vi "audio_crosstalkMeasurement.vi"() -> ()   [LabVIEW 2021, in "audio_crosstalkMeasurement.lvlib"]
uses:
  <vilib>/PDM Acquisition Toolkit/host/Classes/Tasks/PDM Tasks/Controls/Acquisition Mode.ctl
  <vilib>/PDM Acquisition Toolkit/host/Classes/Session/Controls/Logic Levels.ctl
  <vilib>/PDM Acquisition Toolkit/shared/controls/PCM Data Format Configuration.ctl
  <vilib>/PDM Acquisition Toolkit/shared/controls/Digital Edge.ctl
  <vilib>/PDM Acquisition Toolkit/shared/controls/PCM Bit Endianness.ctl
  <vilib>/PDM Acquisition Toolkit/shared/controls/PCM Data Justification.ctl
  <vilib>/PDM Acquisition Toolkit/shared/controls/PCM Frame Sync Control.ctl
  <vilib>/addons/_NISVFA/_Generation/Signal Generation/SV Signal/sv_System Timing Model.ctl
  <vilib>/DAQmx/write.llb/DAQmx Write (Analog 1D Wfm NChan NSamp).vi
  <vilib>/addons/_NISVFA/_Shared subVIs/Common/SVL Set dB Reference (N Ch - 1 Ref).vi
  <vilib>/addons/_NISVFA/_Spectrum Processing/SVFA Unit Conversion (Complex) (1 Ch).vi
  <vilib>/addons/_NISVFA/_Shared subVIs/Common/SVL Set dB Reference (1 Ch).vi
  <vilib>/addons/_NISVFA/_Shared subVIs/Common/svc_Log View for Spectrum (1Ch).vi
  <vilib>/addons/_NISVFA/_Spectrum Processing/SVFA Unit Conversion (1 Ch).vi
  <vilib>/addons/_NISVFA/_Shared subVIs/Common/svc_Complex Datatype Defaults.vi
  <vilib>/addons/_NISVFA/_Shared subVIs/Common/SVL Set dB Reference (variant).vi
  <vilib>/addons/_NISVFA/_Shared subVIs/Common/svc_Unwrap Phase.vi
  <vilib>/addons/_NISVFA/_Shared subVIs/Common/svc_Convert Spectrum Array to dB.vi
  <vilib>/addons/_NISVFA/_Shared subVIs/Common/svc_Spectrum Units.vi
  <vilib>/addons/_NISVFA/_Spectrum Processing/subVIs/svfa_Conversion Utility (spectrum info).vi
  <vilib>/addons/_NISVFA/_Shared subVIs/Common/svc_Format Value (DBL).vi
  <vilib>/addons/_NISVFA/_Shared subVIs/Common/svc_Get Weighting Enum and Labels.vi
  <vilib>/addons/_NISVFA/_Shared subVIs/Common/svc_Engineering Units to Unit Label.vi
  <vilib>/addons/_NISVFA/_Shared subVIs/Common/svc_Surround NonAlpha String with Parentheses.vi
  <vilib>/dlg_ctls.llb/Space Constant.vi
  <vilib>/addons/_NISVFA/_Spectrum Processing/subVIs/svfa_Peak to RMS to Peak2Peak.vi
  <vilib>/addons/_NISVFA/_Spectrum Processing/subVIs/svfa_Mag to Mag2.vi
  <vilib>/addons/_NISVFA/_Spectrum Processing/subVIs/svfa_Linear to dB.vi
  <vilib>/addons/_NISVFA/_Spectrum Processing/subVIs/svfa_dBrefA to dBrefB.vi
  <vilib>/addons/_NISVFA/_Spectrum Processing/subVIs/svfa_Spectrum to Spectral Density.vi
  <vilib>/addons/_NISVFA/_Shared subVIs/Common/svc_Unit Label Lexical Class.vi
  <vilib>/addons/_NISVFA/_Shared subVIs/Common/svc_Window Parameters.vi
  <vilib>/addons/_NISVFA/_Generation/Signal Generation/SV Sinusoid/SV Sinusoid.lvclass
  C:/Program Files/National Instruments/LabVIEW 2021/vi.lib/addons/_NISVFA/_Generation/Signal Generation/SV Signal/SV Signal.lvclass
  <vilib>/DAQmx/create/channels.llb/DAQmx Create Channel (AO-FuncGen).vi
  <vilib>/DAQmx/create/channels.llb/DAQmx Create Channel (AO-Voltage-Basic).vi
  <vilib>/DAQmx/configure/timing.llb/DAQmx Timing (Sample Clock).vi
  <vilib>/addons/_NISVFA/_Generation/Signal Generation/SV Sinusoid/Configure Sine.vi
  <vilib>/addons/_NISVFA/_Generation/Signal Generation/SV Signal/Write Sample Rate.vi
  <vilib>/addons/_NISVFA/_Generation/Signal Generation/SV Signal/Write System Timing Model.vi
  <vilib>/addons/_NISVFA/_Generation/Signal Generation/SV Signal/Write Ramp Parameters.vi
  <vilib>/DAQmx/miscellaneous.llb/DAQmx Fill In Error Info.vi
  <vilib>/PDM Acquisition Toolkit/host/API/Public/Create Tasks/Create PCM Input Task.vi
  <vilib>/PDM Acquisition Toolkit/host/API/Public/Configure/Timing/Configure Timing - PCM Input Slave.vi
  <vilib>/PDM Acquisition Toolkit/host/API/Public/Configure/PDM Channel/Configure Microphone Sensitivity FSPA - PCM Input Task.vi
  <vilib>/PDM Acquisition Toolkit/host/API/Public/Start/Start PCM Input Task.vi
  <vilib>/PDM Acquisition Toolkit/host/API/Public/Read/Read PCM Input Waveform.vi
  <vilib>/addons/_NISVFA/_Shared subVIs/Common/svc_Caller VI Returned in Error Source.vi
  <vilib>/addons/Sound and Vibration/svt_Single Tone Measurements/SVT Crosstalk (Time).vi
  <vilib>/Analysis/4window.llb/window parameters.vi
  <vilib>/Analysis/4window.llb/Window Properties.vi
  <vilib>/Analysis/4window.llb/Window Properties by Name.vi
  <vilib>/PDM Acquisition Toolkit/host/API/Public/Clear/Clear PCM Input Task.vi
  audio_crosstalkMeasurement.lvlib
  <vilib>/addons/Sound and Vibration/svt_Single Tone Measurements/SoundVib_SingleTone.lvlib
  <vilib>/PDM Acquisition Toolkit/host/API/PDM Acquisition Toolkit.lvlib
  <vilib>/PDM Acquisition Toolkit/host/Classes/Tasks/PDM Tasks/PDM Task.lvclass
  <vilib>/PDM Acquisition Toolkit/host/Classes/Session/DecoderSession.lvclass
  <resource>/objmgr/daqmx.rc
  <vilib>/addons/_NISVFA/_Generation/Signal Generation/SV Signal/SV Signal.lvclass
  <vilib>/PDM Acquisition Toolkit/shared/PDM Shared.lvlib
panel:
  in  "Tab Control 2":enum32{"Frequency Domain", "Time Domain"}(tab)=enum."Time Domain"
  out "Spectrum":cluster{"x0":dbl, "dx":dbl, "magnitude":dbl[]}[](graph)
  out "crosstalk":dbl=nan format="%.2f"
  out "Waveform Graph":waveform(dbl)[](graph)
  in  "Tab Control":T1(tab)=enum."Digital Interface"
  in  "Resource name":tag="4468/ao0"
  in  "Frequency":dbl=1000.0 format="%#_6pHz"
  in  "Amplitude":dbl=1.0
  in  "channel list":string="7820\\PCMi 0"
  in  "Sensitivity":dbl=0.34762 format="%#_gFS/Pa"
  in  "Number of words":i32=19200
  in  "Clock rate":u32=12288000 format="%.4pHz"
  in  "Interferer channel":i32
  in  "Victim channel":i32=1
  out "error out":errorcluster
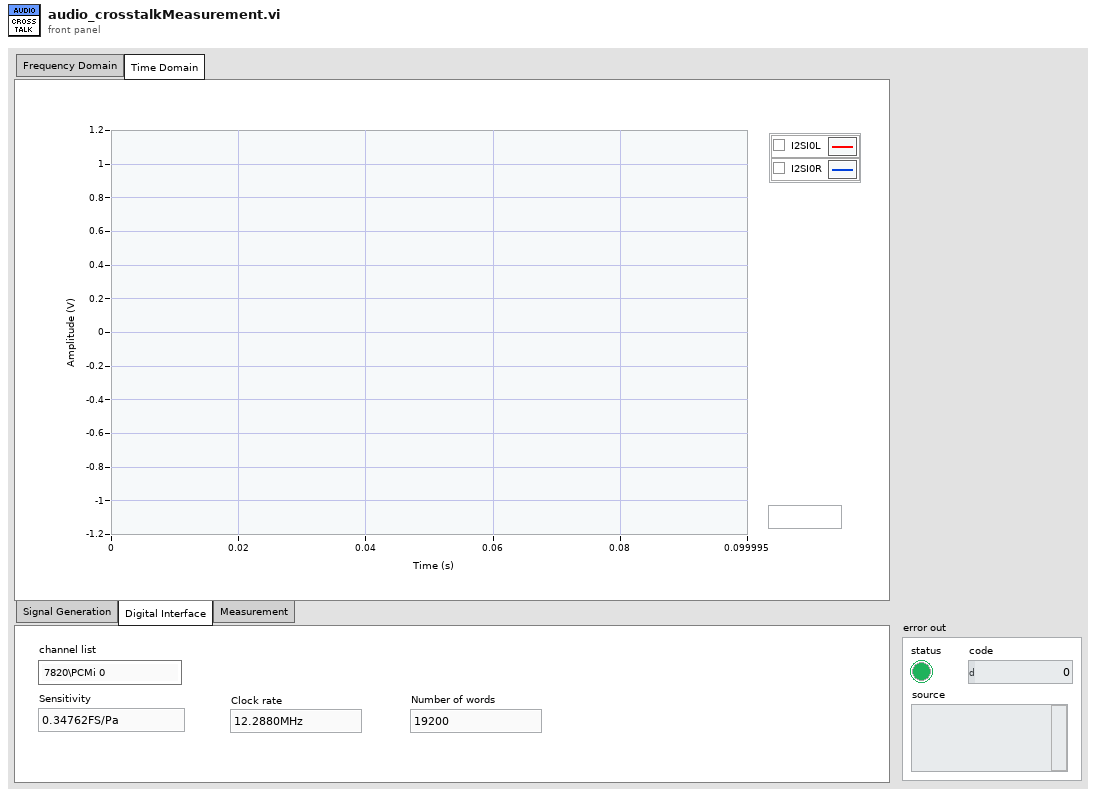
[diagram p1: front panel]
types:
  T1 = enum32{"Signal Generation", "Digital Interface", "Measurement"}
  T2 = typedef "PDM Shared.lvlib/PCM Frame Sync Control.ctl" = cluster{"Frame Length":u16, "Frame Sync Pulse Width":u16, "Bit Clock Edge  Sync":T3}
  T3 = typedef "PDM Shared.lvlib/Digital Edge.ctl" = enum8{"Rising", "Falling"}
  T4 = typedef "PDM Shared.lvlib/PCM Data Format Configuration.ctl" = cluster{"Frame Sync Edge for Channel 0":T3, "Channel Count Per Frame":u8, "Channel Length":u16, "Bit Depth":u8, "Channel 0 Offset":u16, "Endianness":T5, "Data Justification":T6}
  T5 = typedef "PDM Shared.lvlib/PCM Bit Endianness.ctl" = enum16{"MSB First", "LSB First"}
  T6 = typedef "PDM Shared.lvlib/PCM Data Justification.ctl" = enum16{"Left Justified", "Right Justified"}
  T7 = typedef "PDM Acquisition Class Library.lvlib/DecoderSession.lvclass/Logic Levels.ctl" = enum16{"3.3 V", "1.8 V", "1.2 V"}
  T8 = typedef "PDM Acquisition Class Library.lvlib/PDM Task.lvclass/Acquisition Mode.ctl" = enum16{"Finite", "Continuous"}
  T9 = cluster{"linear/dB":enum16{"no change", "linear", "dB"}, "dB reference (0: no change)":dbl, "power/magnitude":enum16{"no change", "power", "magnitude"}, "view":enum16{"no change", "rms", "peak", "peak-peak"}}
  T10 = cluster{"profile":enum16{"Linear", "Half cosine"}, "durations [s]":cluster{"ramp-up":dbl, "transition":dbl, "ramp-down":dbl}}
  T11 = typedef "SV Signal.lvclass/sv_System Timing Model.ctl" = i64
  T12 = typedef "PDM Acquisition Class Library.lvlib/PCM Input Task.lvclass/DVR PCM Input Task.ctl" = refnum<data-value>
  T13 = typedef "svc_Spectrum Info.ctl" = cluster{"channel name":string, "description":string, "x-axis units":T14, "spectral info":cluster{"spectrum type":T15, "linear/dB":enum16{"linear", "dB"}, "window":u16, "window size":i32, "FFT size":i32}, "engineering units":T16, "custom label":string, "dB reference [EU]":dbl, "peak units":enum16{"rms", "peak", "peak-peak"}, "weighting filter":T17, "spectral density?":bool, "unit label":string, "spectrum skewed?":bool, "complimentary spectrum units":T18}
  T14 = typedef "svc_X-Axis Units.ctl" = u16
  T15 = typedef "svc_Spectrum Type.ctl" = enum16{"FFT Spectrum [complex]", "Amplitude [Magnitude]", "Power [Magnitude^2]", "Cross Spectrum [complex]", "Frequency Response [Complex]"}
  T16 = typedef "svc_Engineering Units Text Ring.ctl" = u16
  T17 = typedef "svc_Weighting Filter Text Ring.ctl" = u16
  T18 = typedef "svc_Complimentary Spectrum Units.ctl" = enum16{"none", "radians", "degrees", "cycles", "imaginary"}
  T19 = cluster{"complex spectrum response":cluster{"f0":dbl, "df":dbl, "complex spectrum":cdb[]}, "spectrum info":T13}
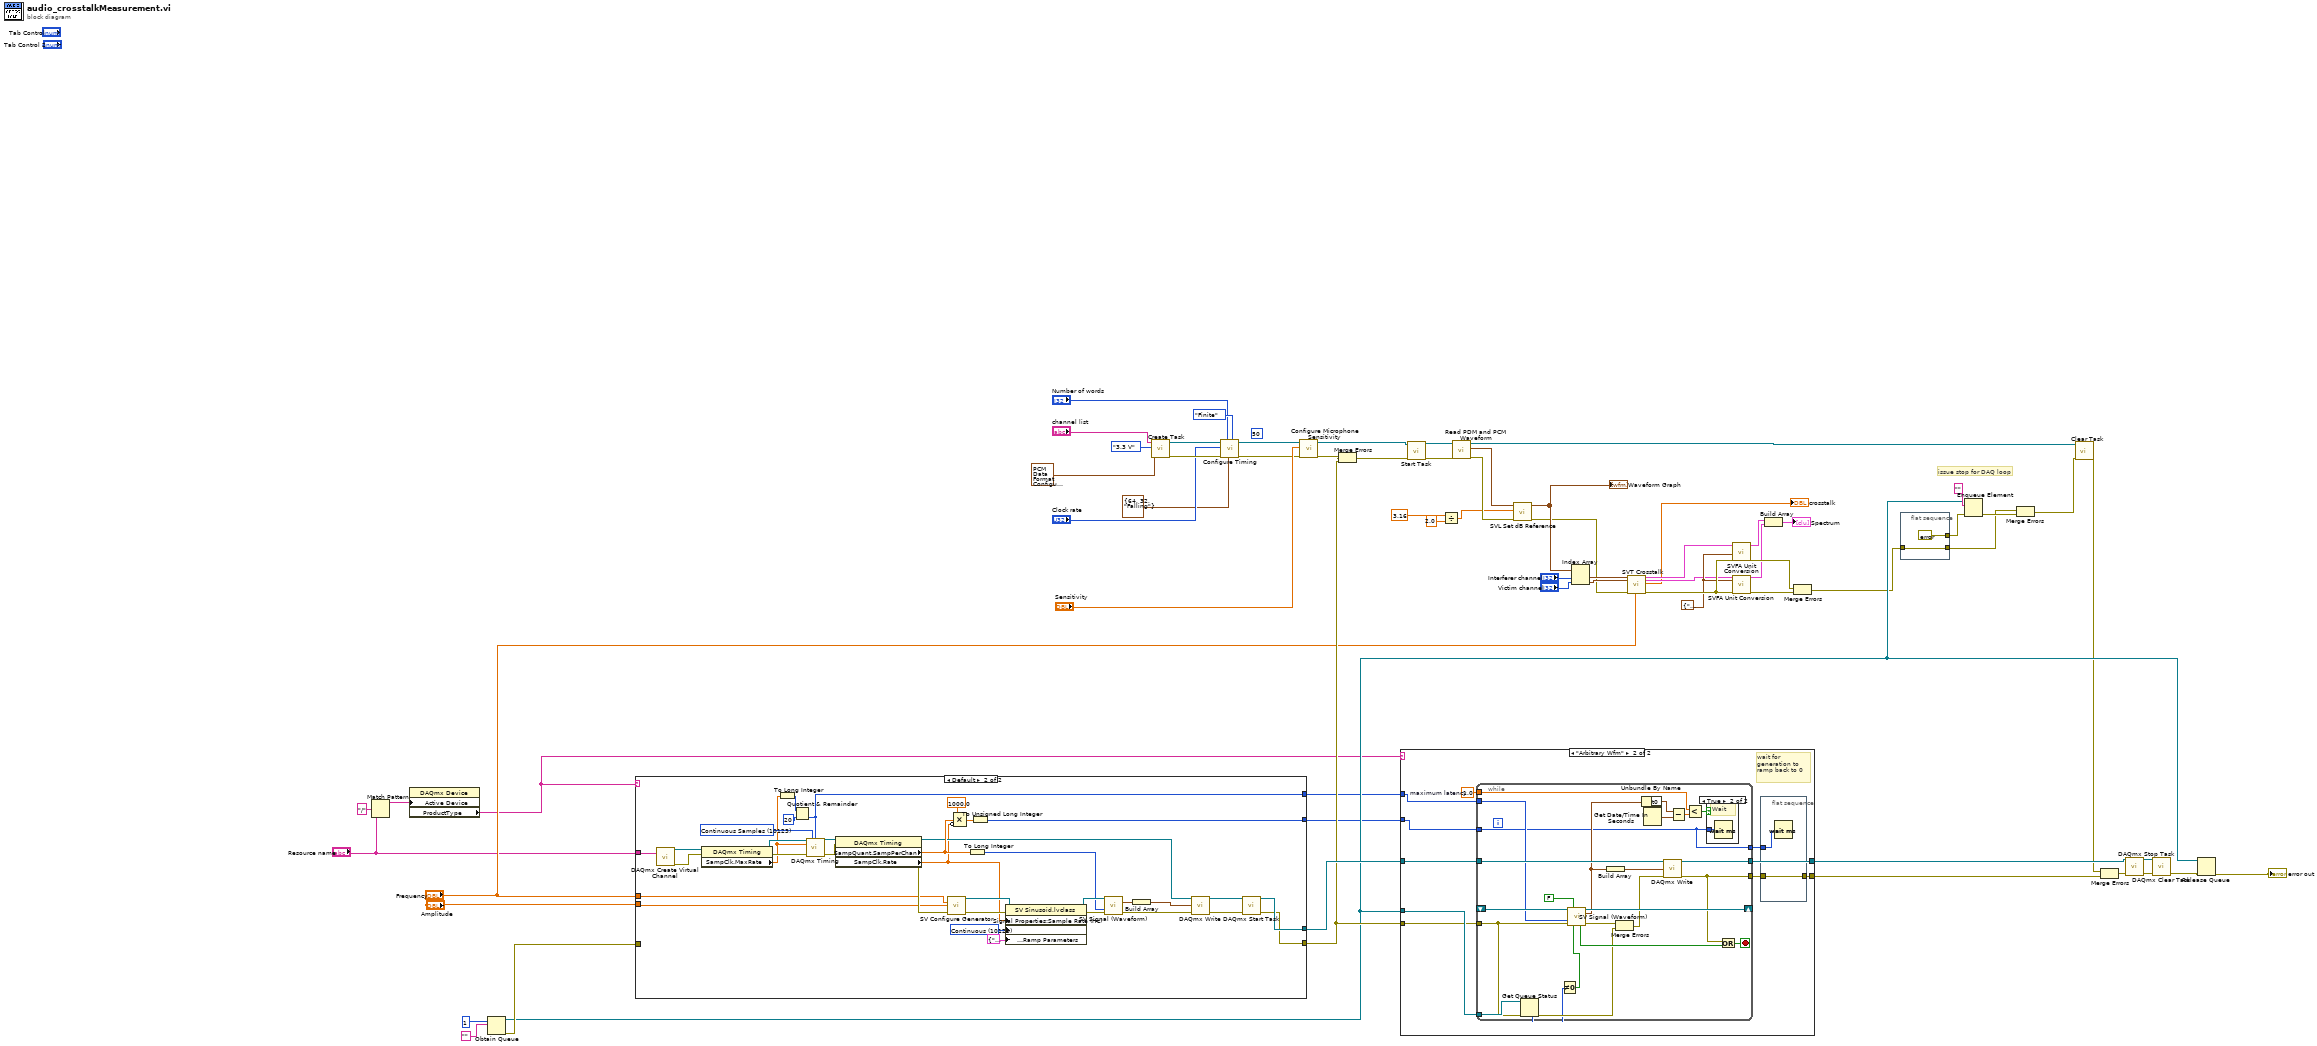
[diagram p0: block diagram]
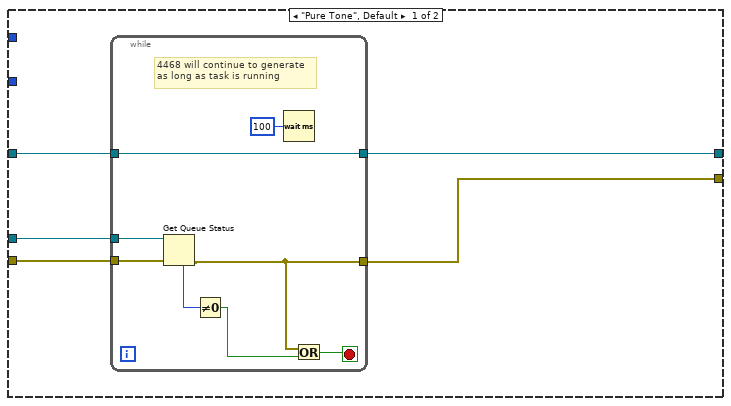
[diagram p2: hidden frame]
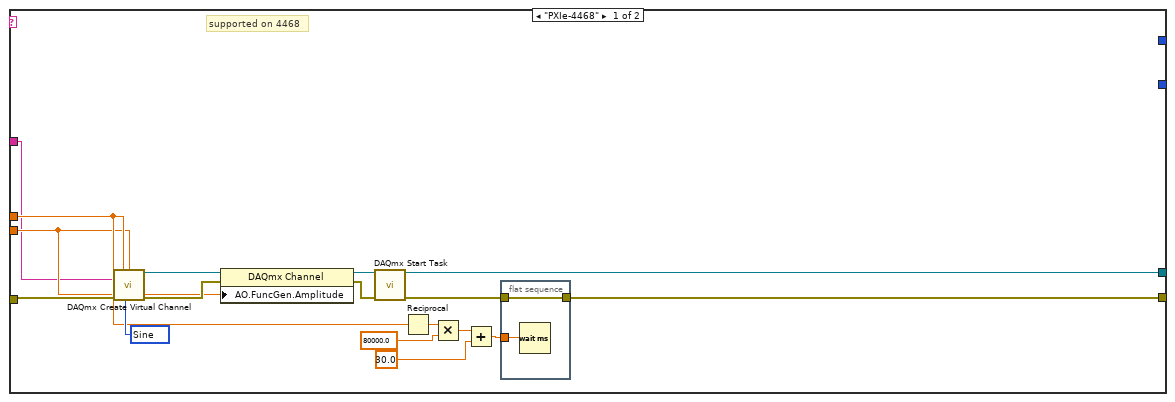
[diagram p4: hidden frame]
diagram:
  (unwired) u8 50 ("data latch at SCK cycle")
  w42 = T9 {"linear/dB"=enum."dB", "dB reference (0: no change)"=0.0, "power/magnitude"=enum."magnitude", "view"=enum."peak"} ("desired scaling")
  # "issue stop for DAQ loop"
  n1 = Match Pattern(string="Resource name", regular expression="/") -> (before substring=w2:string)  [unwired: 1 in, 3 out]
  n2 = property class="DAQmx Device"("Active Device"=w2) -> ("ProductType"=w4:string)  [unwired: 2 in, 2 out]
  n3 = Obtain Queue(max queue size (-1, unlimited)=1, element data type="") -> (queue out=w52:refnum<queue>, error out=w65:errorcluster)  [unwired: 3 in, 1 out]
  n4 = case shown="Default" w4 {
    tunnel: [w72 w93] -> w64
    tunnel: [w71 w92] -> w63
    tunnel: w65 -> [w83 _]
    tunnel: "Frequency" -> [w70 w103]
    tunnel: "Amplitude" -> [w69 w102]
    tunnel: [_ w89] -> w9
    tunnel: [_ w88] -> w10
    tunnel: "Resource name" -> [w68 w87]
    frame "PXIe-4468" {
      w84 = 14751 items=["Sine"=14751, "Triangle"=14752, "Square"=14753, "Sawtooth"=14754] ("type")
      # "supported on 4468"
      n5 = call-poly <vilib>:"DAQmx Create Virtual Channel.vi"("frequency"=w70, "amplitude"=w69, "physical channels"=w68, "type"=w84, "error in"=w83) -> ("task out"=w74:refnum<k21>, "error out"=w73:errorcluster)  [unwired: 9 in]
      n6 = property class="DAQmx Channel"(reference=w74, error in=w73, "AO.FuncGen.Amplitude"=w69) -> (reference out=w76:refnum<k21>, error out=w75:errorcluster)
      n7 = call <vilib>:"DAQmx Start Task.vi"("task/channels in"=w76, "error in"=w75) -> ("task out"=w72:refnum<k21>, "error out"=w82:errorcluster)  [unwired: 12 in]
      n8 = Reciprocal(x=w70) -> (1/x=w81:dbl)
      n9 = Multiply(x=w81, y=80000.0) -> (x*y=w79:dbl)
      n10 = Add(x=w79, y=30.0) -> (x+y=w77:dbl)
      n11 = flat-sequence {
        tunnel: [w86] -> w71
        tunnel: w82 -> [w86]
        tunnel: w77 -> [w85]
        frame #0 {
          n12 = Wait (ms)(milliseconds to wait=w85) -> ()  [unwired: 1 out]
        }
      }
    }
    frame Default {
      w97 = 10123 items=["Finite Samples"=10178, "Continuous Samples"=10123, "Hardware Timed Single Point"=12522] ("sample mode")
      w119 = T11 10123 items=["Finite"=10178, "-"=-1, "Continuous"=10123, "-"=-2, "Settled"=110123, "Averaged"=210123, "Discrete Sweep"=310123, "Continuous Sweep"=410123] ("System Timing Model")
      n13 = call-poly <vilib>:"DAQmx Create Virtual Channel.vi"("physical channels"=w87) -> ("task out"=w98:refnum<k21>, "error out"=w99:errorcluster)  [unwired: 13 in]
      n14 = property class="DAQmx Timing"(reference=w98, error in=w99) -> (reference out=w101:refnum<k21>, error out=w100:errorcluster, "SampClk.MaxRate"=w90:dbl)
      n15 = To Long Integer(number=w90) -> (32bit integer=w91:i32)
      n16 = Quotient & Remainder(x=w91, y=20) -> (floor(x/y)=w89:i32)  [unwired: 1 out]
      n17 = call-poly <vilib>:"DAQmx Timing.vi"("task/channels in"=w101, "sample mode"=w97, "samples per channel"=w89, "rate"=w90, "error in"=w100) -> ("task out"=w95:refnum<k21>, "error out"=w94:errorcluster)  [unwired: 9 in]
      n18 = property class="DAQmx Timing"(reference=w95, error in=w94) -> (reference out=w114:refnum<k21>, error out=w105:errorcluster, "SampQuant.SampPerChan"=w116:dbl, "SampClk.Rate"=w104:dbl)
      n19 = call-poly <vilib>:"SV Configure Generator.vi"("frequency (Hz)"=w103, "amplitude"=w102, "error in (no error)"=w105) -> ("signal configuration"=w120:refnum<class "SV Sinusoid.lvclass">, "error out"=w121:errorcluster)  [unwired: 11 in]
      n20 = Compound Arithmetic op=MULTIPLY(1000.0 ("value"), w116, invert w104) -> (w113:dbl)
      n21 = To Long Integer(number=w116) -> (32bit integer=w115:i32)
      n22 = To Unsigned Long Integer(number=w113) -> (unsigned 32bit integer=w88:u32)
      n23 = property class="SV Sinusoid.lvclass"(reference=w120, error in=w121, "Signal Properties:Sample Rate (Hz)"=w104, "Signal Properties:System Timing Model"=w119, "Signal Properties:Ramps:Ramp Parameters"=T10 {"profile"=enum."Linear", "durations [s]"={"ramp-up"=0.0, "transition"=0.0, "ramp-down"=0.01}} ("Ramp Parameters:All Elements")) -> (reference out=w118:refnum<class "SV Sinusoid.lvclass">, error out=w117:errorcluster)
      n24 = call-dynamic "SV Signal (Waveform).vi"("signal configuration"=w118, "samples"=w115, "error in (no error)"=w117) -> ("output waveform"=w108:waveform(dbl), "error out"=w109:errorcluster)  [unwired: 7 in, 4 out]
      n25 = Build Array(w108) -> (w110:waveform(dbl)[])
      n26 = call-poly <vilib>:"DAQmx Write.vi"("task/channels in"=w114, "data"=w110, "error in"=w109) -> ("task out"=w107:refnum<k21>, "error out"=w106:errorcluster)  [unwired: 10 in, 1 out]
      n27 = call <vilib>:"DAQmx Start Task.vi"("task/channels in"=w107, "error in"=w106) -> ("task out"=w93:refnum<k21>, "error out"=w92:errorcluster)  [unwired: 12 in]
    }
  }
  n28 = call-poly <vilib>:"Create Task.vi"("PCM data configuration"=T4 {"Frame Sync Edge for Channel 0"=enum."Falling", "Channel Count Per Frame"=2, "Channel Length"=32, "Bit Depth"=24, "Channel 0 Offset"=1, "Endianness"=enum."MSB First", "Data Justification"=enum."Left Justified"}, "logic level"=Logic_Levels."3.3 V", "channel list"="channel list") -> ("error out"=w33:errorcluster, "PCM input task out"=w34:T12)  [unwired: 7 in]
  n29 = call-poly <vilib>:"Configure Timing.vi"("acquisition mode"=Acquisition_Mode."Finite", "Frame Sync Clock Control"=T2 {"Frame Length"=64, "Frame Sync Pulse Width"=32, "Bit Clock Edge  Sync"=enum."Falling"}, "number of words per channel"="Number of words", "error in"=w33, "Bit Clock rate"="Clock rate", "PCM input task in"=w34) -> ("error out"=w7:errorcluster, "PCM input task out"=w8:T12)  [unwired: 4 in]
  n30 = call-poly <vilib>:"Configure Microphone Sensitivity.vi"("error in"=w7, "microphone sensitivity (FS/Pa)"="Sensitivity", "PCM input task in"=w8) -> ("error out"=w30:errorcluster, "PCM input task out"=w28:T12)  [unwired: 7 in]
  n31 = Merge Errors(w30, w63) -> (w29:errorcluster)
  n32 = case shown="\"Arbitrary Wfm\"" w4 {
    tunnel: w52 -> [w124 w144]
    tunnel: [w123 w143] -> w60
    tunnel: [w122 w141] -> w12
    tunnel: w64 -> [w126 w140]
    tunnel: w63 -> [w125 w139]
    tunnel: w10 -> [_ w136]
    tunnel: w9 -> [_ w137]
    frame "Pure Tone", Default {
      n33 = while {
        tunnel: w126 -> [w131]
        tunnel: w125 -> [w132]
        tunnel: w124 -> [w133]
        tunnel: [w131] -> w123
        tunnel: [w127] -> w122
        stop <- w130 stop-if-true
        # "4468 will continue to generate as long as task is running"
        n34 = Get Queue Status(queue=w133, error in (no error)=w132) -> (error out=w127:errorcluster, # elements in queue=w134:i32)  [unwired: 1 in, 6 out]
        n35 = Not Equal To 0?(x=w134) -> (x != 0?=w129:bool)
        n36 = Wait (ms)(milliseconds to wait=u32 100) -> ()  [unwired: 1 out]
        n37 = Or(x=w127, y=w129) -> (x .or. y?=w130:bool)
      }
    }
    frame "Arbitrary Wfm" {
      w138 = 1.0  # maximum latency
      # "wait for generation to ramp back to 0"
      n38 = while {
        tunnel: w139 -> [w149]
        shift-right: [w169] -> _
        shift-left: _ -> [w170]
        tunnel: w140 -> [w166]
        tunnel: [w165] -> w143
        tunnel: [w164] -> w142
        tunnel: w138 -> [w160]
        tunnel: w144 -> [w154]
        tunnel: w137 -> [w148]
        tunnel: w136 -> [w147]
        tunnel: [w147] -> w135
        stop <- w168 stop-if-true
        n39 = Get Queue Status(queue=w154, error in (no error)=w149) -> (error out=w152:errorcluster, # elements in queue=w151:i32)  [unwired: 1 in, 6 out]
        n40 = Not Equal To 0?(x=w151) -> (x != 0?=w153:bool)
        n41 = call-dynamic "SV Signal (Waveform).vi"("signal configuration"=w170, "reset"=FALSE, "samples"=w148, "error in (no error)"=w149, "stop"=w153) -> ("signal configuration"=w169:refnum<class "SV Sinusoid.lvclass">, "output waveform"=w158:waveform(dbl), "done"=w167:bool, "error out"=w156:errorcluster)  [unwired: 5 in, 2 out]
        n42 = Build Array(w158) -> (w157:waveform(dbl)[])
        n43 = Merge Errors(w156, w152) -> (w155:errorcluster)
        n44 = Unbundle By Name(w158) -> ("t0"=w163:timestamp)
        n45 = Get Date/Time In Seconds() -> (seconds since 1Jan1904=w162:timestamp)
        n46 = call-poly <vilib>:"DAQmx Write.vi"("task/channels in"=w166, "data"=w157, "error in"=w155) -> ("task out"=w165:refnum<k21>, "error out"=w164:errorcluster)  [unwired: 10 in, 1 out]
        n47 = Subtract(x=w163, y=w162) -> (x-y=w161:dbl)
        n48 = Less?(x=w160, y=w161) -> (x < y?=w159:bool)
        n49 = case shown="True" w159 {
          tunnel: w147 -> [_ w171]
          frame False {
          }
          frame True {
            # "Wait"
            n50 = Wait (ms)(milliseconds to wait=w171) -> ()  [unwired: 1 out]
          }
        }
        n51 = Or(x=w164, y=w167) -> (x .or. y?=w168:bool)
      }
      n52 = flat-sequence {
        tunnel: w142 -> [w146]
        tunnel: [w146] -> w141
        tunnel: w135 -> [w145]
        frame #0 {
          n53 = Wait (ms)(milliseconds to wait=w145) -> ()  [unwired: 1 out]
        }
      }
    }
  }
  n54 = call-poly <vilib>:"Start Task.vi"("error in"=w29, "PCM input task in"=w28) -> ("error out"=w26:errorcluster, "PCM input task out"=w27:T12)  [unwired: 8 in]
  n55 = Divide(x=3.16, y=2.0) -> (x/y=w15:dbl)
  n56 = call-poly <vilib>:"Read PDM and PCM Waveform.vi"("error in"=w26, "PCM input task In"=w27) -> ("error out"=w25:errorcluster, "PCM waveforms"=w24:waveform(dbl)[], "PCM input task out"=w22:T12)  [unwired: 4 in, 3 out]
  n57 = call-poly <vilib>:"SVL Set dB Reference.vi"("error in (no error)"=w25, "dB reference [EU]"=w15, "scaled signals in [EU]"=w24) -> ("error out"=w35:errorcluster, "scaled signals out [EU]"=w36:waveform(dbl)[])  [unwired: 7 in]
  "Waveform Graph" <- w36
  n58 = Index Array(array=w36, index #1="Interferer channel", index #2="Victim channel") -> (element #1=w49:waveform(dbl), element #2=w48:waveform(dbl))
  n59 = call-poly <vilib>:"SVT Crosstalk.vi"("stimulus signal X [EUx]"=w49, "idle-channel response signal Y [EUy]"=w48, "error in (no error)"=w35, "expected fundamental frequency [Hz]"="Frequency") -> ("complex spectrum\nstimulus X"=w47:T19, "complex spectrum\nidle-channel response Y"=w41:T19, "crosstalk"=→"crosstalk":dbl, "error out"=w46:errorcluster)  [unwired: 8 in, 4 out]
  n60 = call-poly <vilib>:"SVFA Unit Conversion.vi"("complex spectrum"=w47, "desired scaling"=w42, "error in (no error)"=w46) -> ("converted spectrum"=w40:cluster{"x0":dbl, "dx":dbl, "magnitude":dbl[]}, "error out"=w44:errorcluster)  [unwired: 11 in, 4 out]
  n61 = call-poly <vilib>:"SVFA Unit Conversion.vi"("complex spectrum"=w41, "desired scaling"=w42, "error in (no error)"=w46) -> ("converted spectrum"=w39:cluster{"x0":dbl, "dx":dbl, "magnitude":dbl[]}, "error out"=w45:errorcluster)  [unwired: 11 in, 4 out]
  n62 = Build Array(w40, w39) -> (→"Spectrum":cluster{"x0":dbl, "dx":dbl, "magnitude":dbl[]}[])
  n63 = Merge Errors(w44, w45) -> (w43:errorcluster)
  n64 = flat-sequence {
    tunnel: w43 -> [w172]
    tunnel: [errorcluster {"status"=FALSE, "code"=0, "source"=""} ("error in (no error)")] -> w57
    tunnel: [w172] -> w55
    frame #0 {
    }
  }
  n65 = Enqueue Element(queue=w52, element="", error in (no error)=w57) -> (error out=w56:errorcluster)  [unwired: 1 in, 2 out]
  n66 = Merge Errors(w55, w56) -> (w23:errorcluster)
  n67 = call-poly <vilib>:"Clear Task.vi"("error in"=w23, "PCM input task in"=w22) -> ("error out"=w13:errorcluster)  [unwired: 9 in]
  n68 = Merge Errors(w13, w12) -> (w59:errorcluster)
  n69 = call <vilib>:"DAQmx Stop Task.vi"("task/channels in"=w60, "error in"=w59) -> ("task out"=w62:refnum<k21>, "error out"=w61:errorcluster)  [unwired: 12 in]
  n70 = call <vilib>:"DAQmx Clear Task.vi"("task in"=w62, "error in"=w61) -> ("error out"=w54:errorcluster)  [unwired: 13 in]
  n71 = Release Queue(queue=w52, error in (no error)=w54) -> (error out=→"error out":errorcluster)  [unwired: 1 in, 2 out]
